vi "Command Status.vi"(8 "error in (no error)":errorcluster, 11 "GUI Manager Module in":refnum<class "GUI Manager Module.lvclass">) -> (0 "error out":errorcluster, 1 "Cmd Active":bool, 2 "Cmd Status":cluster{u32, string}, 3 "GUI Manager Module out":refnum<class "GUI Manager Module.lvclass">)   [LabVIEW 2020, in "VolatusGUI.lvlib" / "GUI Manager Module.lvclass"]
uses:
  GUI Manager Module.lvclass
  GUI Manager Module.lvclass/GUI Manager Module.ctl
  Volatus/Module/Module.lvclass
  Volatus/VolatusAPI/VolatusAPI.lvclass
  C:/dev/lv20CE/relink/lv-volatus/Volatus/Module/Module.lvclass
  C:/dev/lv20CE/relink/lv-volatus/VolatusGUI/GUI Manager Module/GUI Manager Module.lvclass
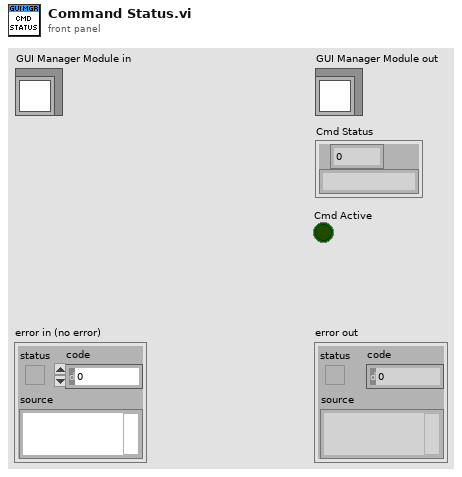
[diagram p1: front panel]
types:
  T1 = typedef "Vecto.lvlib/Connected Status.ctl" = enum16{"Inactive", "Disconnected", "Connected", "Bad Config", "Not Allowed", "Server"}
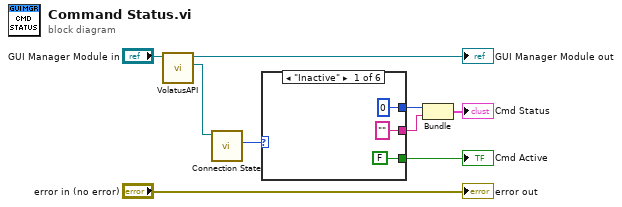
[diagram p0: block diagram]
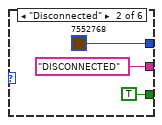
[diagram p2: hidden frame]
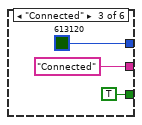
[diagram p3: hidden frame]
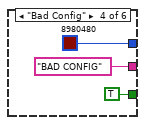
[diagram p4: hidden frame]
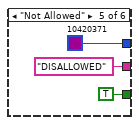
[diagram p5: hidden frame]
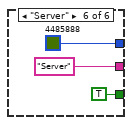
[diagram p6: hidden frame]
diagram:
  n1 = call "VolatusAPI.vi"("Module in"="GUI Manager Module in") -> ("VolatusAPI"=w3:refnum<class "VolatusAPI.lvclass">, "Module out"=→"GUI Manager Module out":refnum<class "GUI Manager Module.lvclass">)  [unwired: 9 in]
  n2 = call "Connection State.vi"("VolatusAPI in"=w3) -> ("Connected Status"=w8:T1)  [unwired: 8 in, 2 out]
  n3 = case shown="\"Inactive\"" w8 {
    tunnel: ["" "DISCONNECTED" "Connected" "BAD CONFIG" "DISALLOWED" "Server"] -> w6
    tunnel: [u32 0 u32 7552768 u32 613120 u32 8980480 u32 10420371 u32 4485888] -> w7
    tunnel: [FALSE TRUE TRUE TRUE TRUE TRUE] -> w1
    frame "Inactive" {
    }
    frame "Disconnected" {
    }
    frame "Connected" {
    }
    frame "Bad Config" {
    }
    frame "Not Allowed" {
    }
    frame "Server" {
    }
  }
  "Cmd Active" <- w1
  n4 = Bundle(w7, w6) -> (→"Cmd Status":cluster{u32, string})  [unwired: 1 in]
  "error out" <- "error in (no error)"
